vi "Gyro_State_Art.vi"(0 "reset integrator":bool, 1 "[ESC]":bool) -> (6 "Linear Acceleration [LSB/sec^2]":cluster{i16, i16, i16}(graph), 7 "Z displacement":dbl format="%#_5g", 8 "X acc":i16, 9 "Y displacement":dbl format="%#_5g", 10 "Y acc":i16, 11 "X displacement":dbl format="%#_5g", 12 "Angular rate [LSB/sec]":cluster{dbl, dbl, dbl}(graph), 13 "Y rot rate":i16, 14 "Z acc":i16, 15 "Z rot rate":i16, 16 "Temp":i16, 17 "Angular displacement [LSB]":T1(graph), 18 "X rot rate":i16)   [LabVIEW 2017]
uses:
  <vilib>/myRIO/Instrument Drivers/Onboard IO/I2C/typedefs/I2C User Configuration.ctl
  <vilib>/myRIO/Instrument Drivers/Onboard IO/I2C/typedefs/I2C Transfer Rate.ctl
  <vilib>/Platform/TimedLoop/XDataNode/timing_clust.ctl
  <vilib>/Platform/TimedLoop/XDataNode/nitl_modes.ctl
  <vilib>/Platform/TimedLoop/XDataNode/wakeup.ctl
  <vilib>/myRIO/Instrument Drivers/Onboard IO/PWM/typedefs/PWM Reference.ctl
  <vilib>/myRIO/Common/Instrument Driver Framework/Utilities/typedefs/myRIO Generic Hardware Reference.ctl
  <vilib>/myRIO/Common/Instrument Driver Framework/Utilities/typedefs/Hardware Version Enum.ctl
  <vilib>/myRIO/Common/Instrument Driver Framework/Utilities/typedefs/myRIO v1.0 Reference.ctl
  <vilib>/myRIO/Common/Instrument Driver Framework/Utilities/typedefs/Generic FPGA Reference.ctl
  <vilib>/myRIO/Common/Instrument Driver Framework/myRIO v1.0/PWM/typedefs/PWM Channels Enum.ctl
  <vilib>/myRIO/Instrument Drivers/Onboard IO/PWM/typedefs/PWM Configuration.ctl
  <vilib>/userdefined/High Color/nirio_resource_hc.ctl
  <vilib>/myRIO/Common/Instrument Driver Framework/Utilities/vis/Is FPGA Ref Available.vi
  <vilib>/myRIO/Common/Instrument Driver Framework/myRIO v1.0/PWM/vis/myRIO v1.1 Open PWM.vi
  <vilib>/myRIO/Instrument Drivers/Onboard IO/PWM/vis/Set Duty Cycle and Frequency.vi
  <vilib>/myRIO/Common/Instrument Driver Framework/myRIO v1.0/DIO/vis/myRIO v1.1 Open DIO.vi
  <vilib>/myRIO/Common/Instrument Driver Framework/myRIO v1.0/I2C/vis/myRIO v1.1 Open I2C.vi
  <vilib>/myRIO/Common/Instrument Driver Framework/Utilities/vis/Validate Channels.vi
  <vilib>/myRIO/Common/Instrument Driver Framework/myRIO v1.0/PWM/vis/myRIO v1.0 Reserve PWM.vi
  <vilib>/myRIO/Common/Instrument Driver Framework/myRIO v1.0/UART/vis/myRIO v1.0 Close UART.vi
  <vilib>/myRIO/Common/Instrument Driver Framework/myRIO v1.0/DIO/vis/myRIO v1.0 Reserve DIO.vi
  <vilib>/myRIO/Common/Instrument Driver Framework/myRIO v1.0/I2C/vis/myRIO v1.0 Reserve I2C.vi
  <vilib>/myRIO/Common/Instrument Driver Framework/myRIO v1.0/PWM/vis/myRIO v1.0 Build MUX Configuration PWM.vi
  <vilib>/myRIO/Common/Instrument Driver Framework/myRIO v1.0/Resource Manager/vis/myRIO v1.0 Reserve Channel List.vi
  <vilib>/myRIO/Common/Instrument Driver Framework/myRIO v1.0/DIO/vis/myRIO v1.0 Build MUX Configuration DIO.vi
  <vilib>/myRIO/Common/Instrument Driver Framework/myRIO v1.0/I2C/vis/myRIO v1.0 Build MUX Configuration I2C.vi
  <vilib>/myRIO/Common/Instrument Driver Framework/myRIO v1.0/Resource Manager/vis/myRIO v1.0 Create Configuration List.vi
  <vilib>/myRIO/Common/Instrument Driver Framework/myRIO v1.0/Resource Manager/vis/myRIO v1.0 Reserve Channel.vi
  <vilib>/myRIO/Common/Instrument Driver Framework/myRIO v1.0/Resource Manager/vis/myRIO v1.0 Unreserve Channel.vi
  <vilib>/myRIO/Common/Instrument Driver Framework/myRIO v1.0/Resource Manager/vis/myRIO v1.0 Build Mutex Name.vi
  <vilib>/Utility/VariantDataType/GetNumericInfo.vi
  <vilib>/Utility/error.llb/Error Cluster From Error Code.vi
  <vilib>/myRIO/Common/Instrument Driver Framework/myRIO v1.0/myRIO v1.1 Open.vi
  <vilib>/myRIO/Common/Instrument Driver Framework/Utilities/vis/IO Manager.vi
  <vilib>/myRIO/Common/Instrument Driver Framework/Utilities/vis/Configuration Manager.vi
  <vilib>/myRIO/Common/Instrument Driver Framework/myRIO v1.0/Resource Manager/vis/myRIO v1.0 Configure IO.vi
  <vilib>/myRIO/Common/Instrument Driver Framework/myRIO v1.0/myRIO v1.0 Close.vi
  <vilib>/myRIO/Common/Instrument Driver Framework/myRIO v1.0/I2C/vis/myRIO v1.0 Configure I2C.vi
  <vilib>/myRIO/Common/Instrument Driver Framework/myRIO v1.0/I2C/vis/myRIO v1.0 Write I2C.vi
  <vilib>/myRIO/Common/Instrument Driver Framework/myRIO v1.0/PWM/vis/myRIO v1.0 Write PWM.vi
  <vilib>/myRIO/Common/Instrument Driver Framework/myRIO v1.0/DIO/vis/myRIO v1.0 Read DIO.vi
  <vilib>/myRIO/Common/Instrument Driver Framework/myRIO v1.0/I2C/vis/myRIO v1.0 Read I2C.vi
  <vilib>/myRIO/Common/Instrument Driver Framework/Utilities/vis/FPGA Ref Manager.vi
  <vilib>/myRIO/Common/Instrument Driver Framework/myRIO v1.0/myRIO v1.0 Reset FPGA.vi
  <vilib>/myRIO/Common/Instrument Driver Framework/myRIO v1.0/IRQ/vis/myRIO v1.0 IRQ Info FGV.vi
  <vilib>/myRIO/Common/Instrument Driver Framework/myRIO v1.0/IRQ/vis/myRIO v1.0 Timer IRQ Info FGV.vi
  <vilib>/myRIO/Common/Instrument Driver Framework/myRIO v1.0/IRQ/vis/myRIO v1.0 ISR Agent.vi
  <vilib>/Platform/TimedLoop/XDataNode/XDataNode.xnode
  <vilib>/myRIO/Express VI/Onboard IO/PWM/PWM Express VI.xnode
  <vilib>/myRIO/Instrument Drivers/Onboard IO/PWM/vis/myRIO PWM Open.xnode
  <vilib>/myRIO/Instrument Drivers/Utilities/Utilities.lvlib
  <vilib>/myRIO/Instrument Drivers/Onboard IO/I2C/I2C.lvlib
  <vilib>/myRIO/Instrument Drivers/Onboard IO/DIO/DIO.lvlib
  <vilib>/Platform/TimedLoop/XDataNode/XDNodeRunTimeDep.lvlib
  <vilib>/ptbypt/NI_PtbyPt.lvlib
  <vilib>/myRIO/Instrument Drivers/Onboard IO/PWM/PWM.lvlib
panel:
  in  "Brushless controller Duty Cycle":dbl(slide)=0.05 scale=0.05..0.1 scale format="%#_6f"
  in  "Duty Cycle MCC2 : Faixa de operação":dbl(slide) scale=0.0..1.0
  in  "Controle sentido M2":bool
  in  "Duty Cycle MCC1 : Faixa de operação":dbl(slide) scale=0.0..1.0
  in  "Ligar (StandBy)":bool
  in  "Controle sentido M1":bool
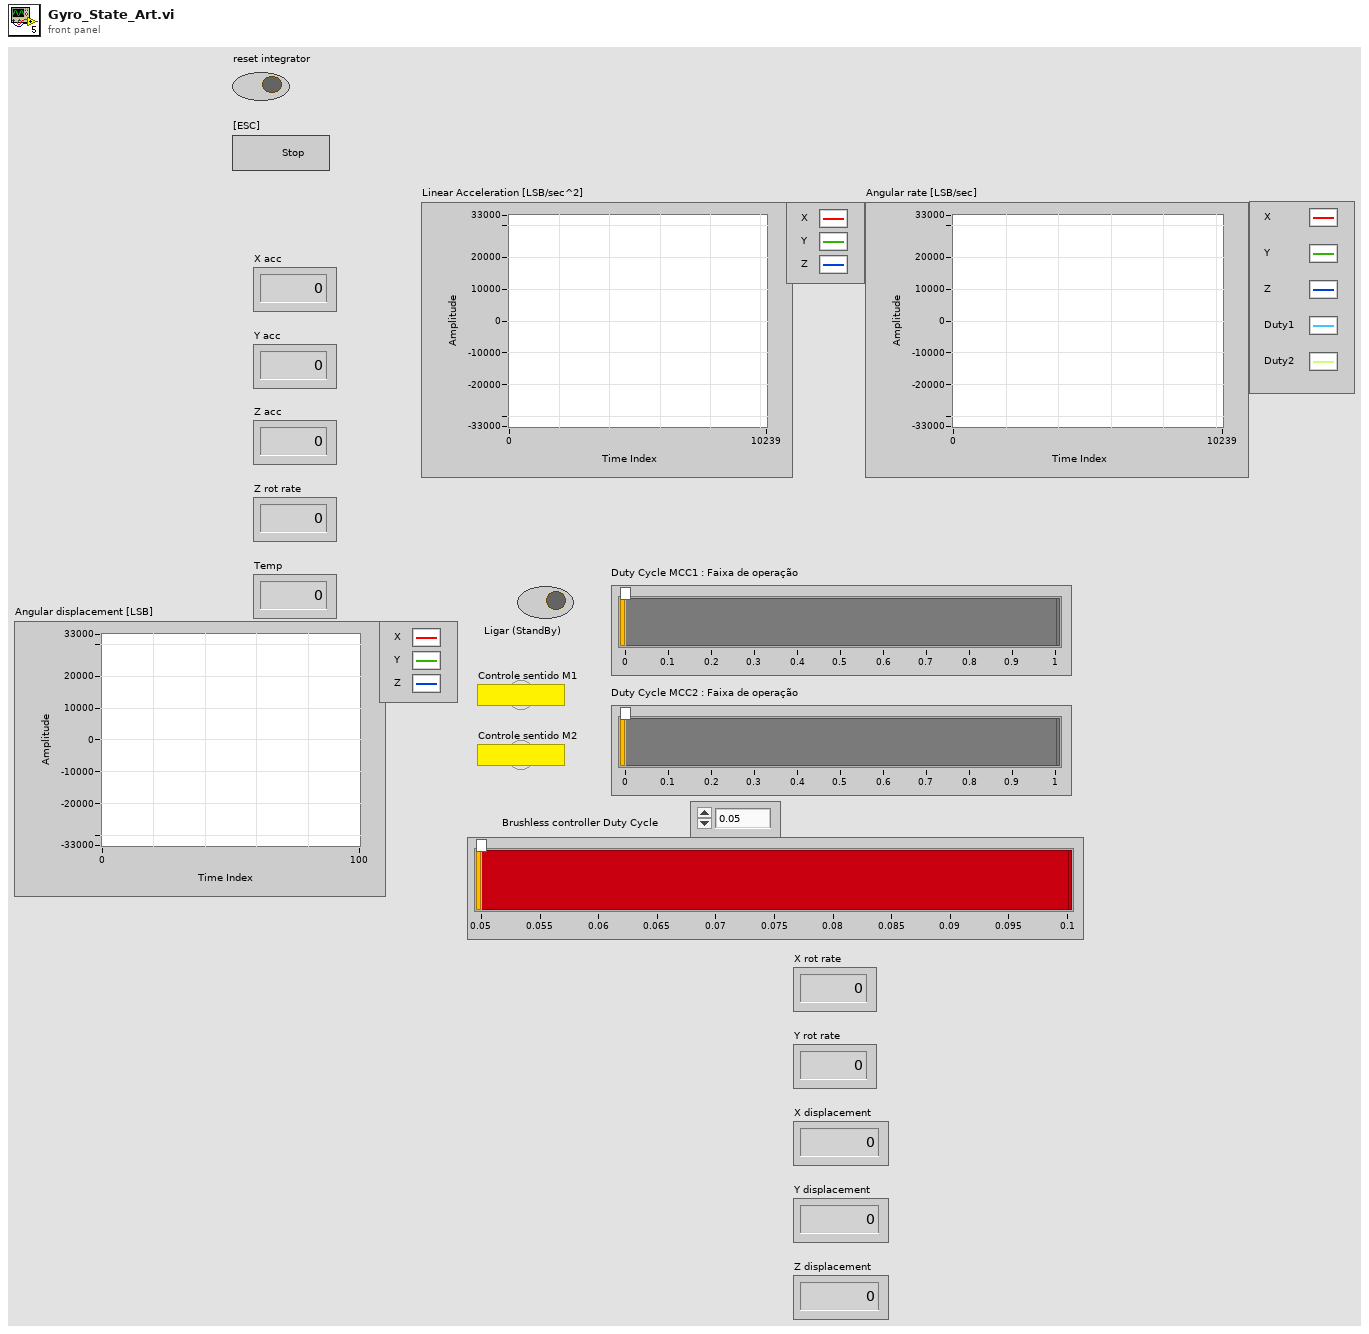
[diagram p1: front panel]
types:
  T1 = cluster{"integral x(t)":dbl, "integral x(t)":dbl, "integral x(t)":dbl}
  T2 = typedef "I2C.lvlib/I2C User Configuration.ctl" = cluster{"I2C Transfer Rate":T3}
  T3 = typedef "I2C.lvlib/I2C Transfer Rate.ctl" = enum16{"Standard mode (100 kbps)", "Fast mode (400 kbps)"}
  T4 = typedef "I2C.lvlib/I2C Reference.ctl" = cluster{"myRIO Reference":T5, "I2C Channels Enum":T9, "I2C Configuration":T10}
  T5 = typedef "myRIO Generic Hardware Reference.ctl" = cluster{"myRIO Model":T6, "myRIO Hardware Reference":T7}
  T6 = typedef "Hardware Version Enum.ctl" = enum16{"Unknown", "myRIO-1900", "myRIO-1950", "roboRIO", "NI ELVIS RIO CM"}
  T7 = typedef "myRIO v1.0 Reference.ctl" = cluster{"Generic FPGA Reference":T8, "Allow multiple opens":bool}
  T8 = typedef "Generic FPGA Reference.ctl" = refnum<k20>
  T9 = typedef "I2C Channels Enum.ctl" = enum16{"Not Connected", "A/I2C", "B/I2C", "I2C/I2C"}
  T10 = typedef "I2C.lvlib/I2C Configuration.ctl" = cluster{"I2C Transfer Rate":T3}
  T11 = typedef "DIO.lvlib/DIO Reference.ctl" = cluster{"myRIO Reference":T5, "DIO Channels List":T12}
  T12 = typedef "DIO Channels List.ctl" = T13[]
  T13 = typedef "DIO Channels Enum.ctl" = enum16{"Not Connected", "C/DIO0", "C/DIO1", "C/DIO2", "C/DIO3", "C/DIO4", "C/DIO5", "C/DIO6", "C/DIO7", "A/DIO0", "A/DIO1", "A/DIO2", "A/DIO3", "A/DIO4", "A/DIO5", "A/DIO6", "A/DIO7", "A/DIO8", "A/DIO9", "A/DIO10", "A/DIO11", "A/DIO12", "A/DIO13", "A/DIO14", "A/DIO15", "B/DIO0", "B/DIO1", "B/DIO2", "B/DIO3", "B/DIO4", "B/DIO5", "B/DIO6", "B/DIO7", "B/DIO8", "B/DIO9", "B/DIO10", "B/DIO11", "B/DIO12", "B/DIO13", "B/DIO14", "B/DIO15", "LED0", "LED1", "LED2", "LED3", "Button0", "DIO/DIO0", "DIO/DIO1", "DIO/DIO2", "DIO/DIO3", "DIO/DIO4", "DIO/DIO5", "DIO/DIO6", "DIO/DIO7", "DIO/DIO8", "DIO/DIO9", "SPI/CS0", "SPI/CS1", "SPI/CS2", "SPI/CS3", "LED RADIO (Green)", "LED RADIO (Red)", "LED COMM (Green)", "LED COMM (Red)", "LED MODE (Green)", "LED MODE (Red)"}
  T14 = typedef "XDNodeRunTimeDep.lvlib/timing_clust.ctl" = cluster{"Expected End [f-1]":u64, "Actual End [f-1]":u64, "Finished Late? [f-1]":bool, "Expected End [i-1]":u64, "Actual End [i-1]":u64, "Finished Late? [i-1]":bool, "Expected Start [i]":u64, "Actual Start [i]":u64, "Expected Start [f]":u64, "Actual Start [f]":u64, "Source Name":string, "Structure Name":string, "Period":i64, "Deadline":i64, "Offset":i64, "Start":i64, "Priority":i32, "Timeout":i32, "Mode":T15, "Wakeup Reason":T16, "Error":errorcluster, "Source Type":string, "Secondary Source Type":string, "Global End Time":u64, "Global Start Time":u64, "Frame Duration":u64, "Iteration Duration":u64, "Assigned CPU":i32, "I/O Scan Engine Mode":u32}
  T15 = typedef "XDNodeRunTimeDep.lvlib/nitl_modes.ctl" = enum32{"No Change", "Process missed periods, maintain original phase", "Discard missed periods, maintain original phase", "Process missed periods, ignore original phase", "Discard missed periods, ignore original phase"}
  T16 = typedef "XDNodeRunTimeDep.lvlib/wakeup.ctl" = enum32{"Normal", "Aborted", "Asynchronous wakeup", "Timing source error", "Timed loop error", "Timeout"}
  T17 = typedef "PWM.lvlib/PWM Reference.ctl" = cluster{"myRIO Reference":T5, "PWM Channels Enum":T18, "PWM Configuration":T19}
  T18 = typedef "PWM Channels Enum.ctl" = enum16{"Not Connected", "C/PWM0", "C/PWM1", "A/PWM0", "A/PWM1", "A/PWM2", "B/PWM0", "B/PWM1", "B/PWM2", "PWM/PWM0", "PWM/PWM1", "PWM/PWM2", "PWM/PWM3", "PWM/PWM4", "PWM/PWM5", "PWM/PWM6", "PWM/PWM7", "PWM/PWM8", "PWM/PWM9"}
  T19 = typedef "PWM.lvlib/PWM Configuration.ctl" = cluster{"Frequency":dbl, "Duty Cycle":dbl}
  T20 = typedef "nirio_resource_hc.ctl" = tag
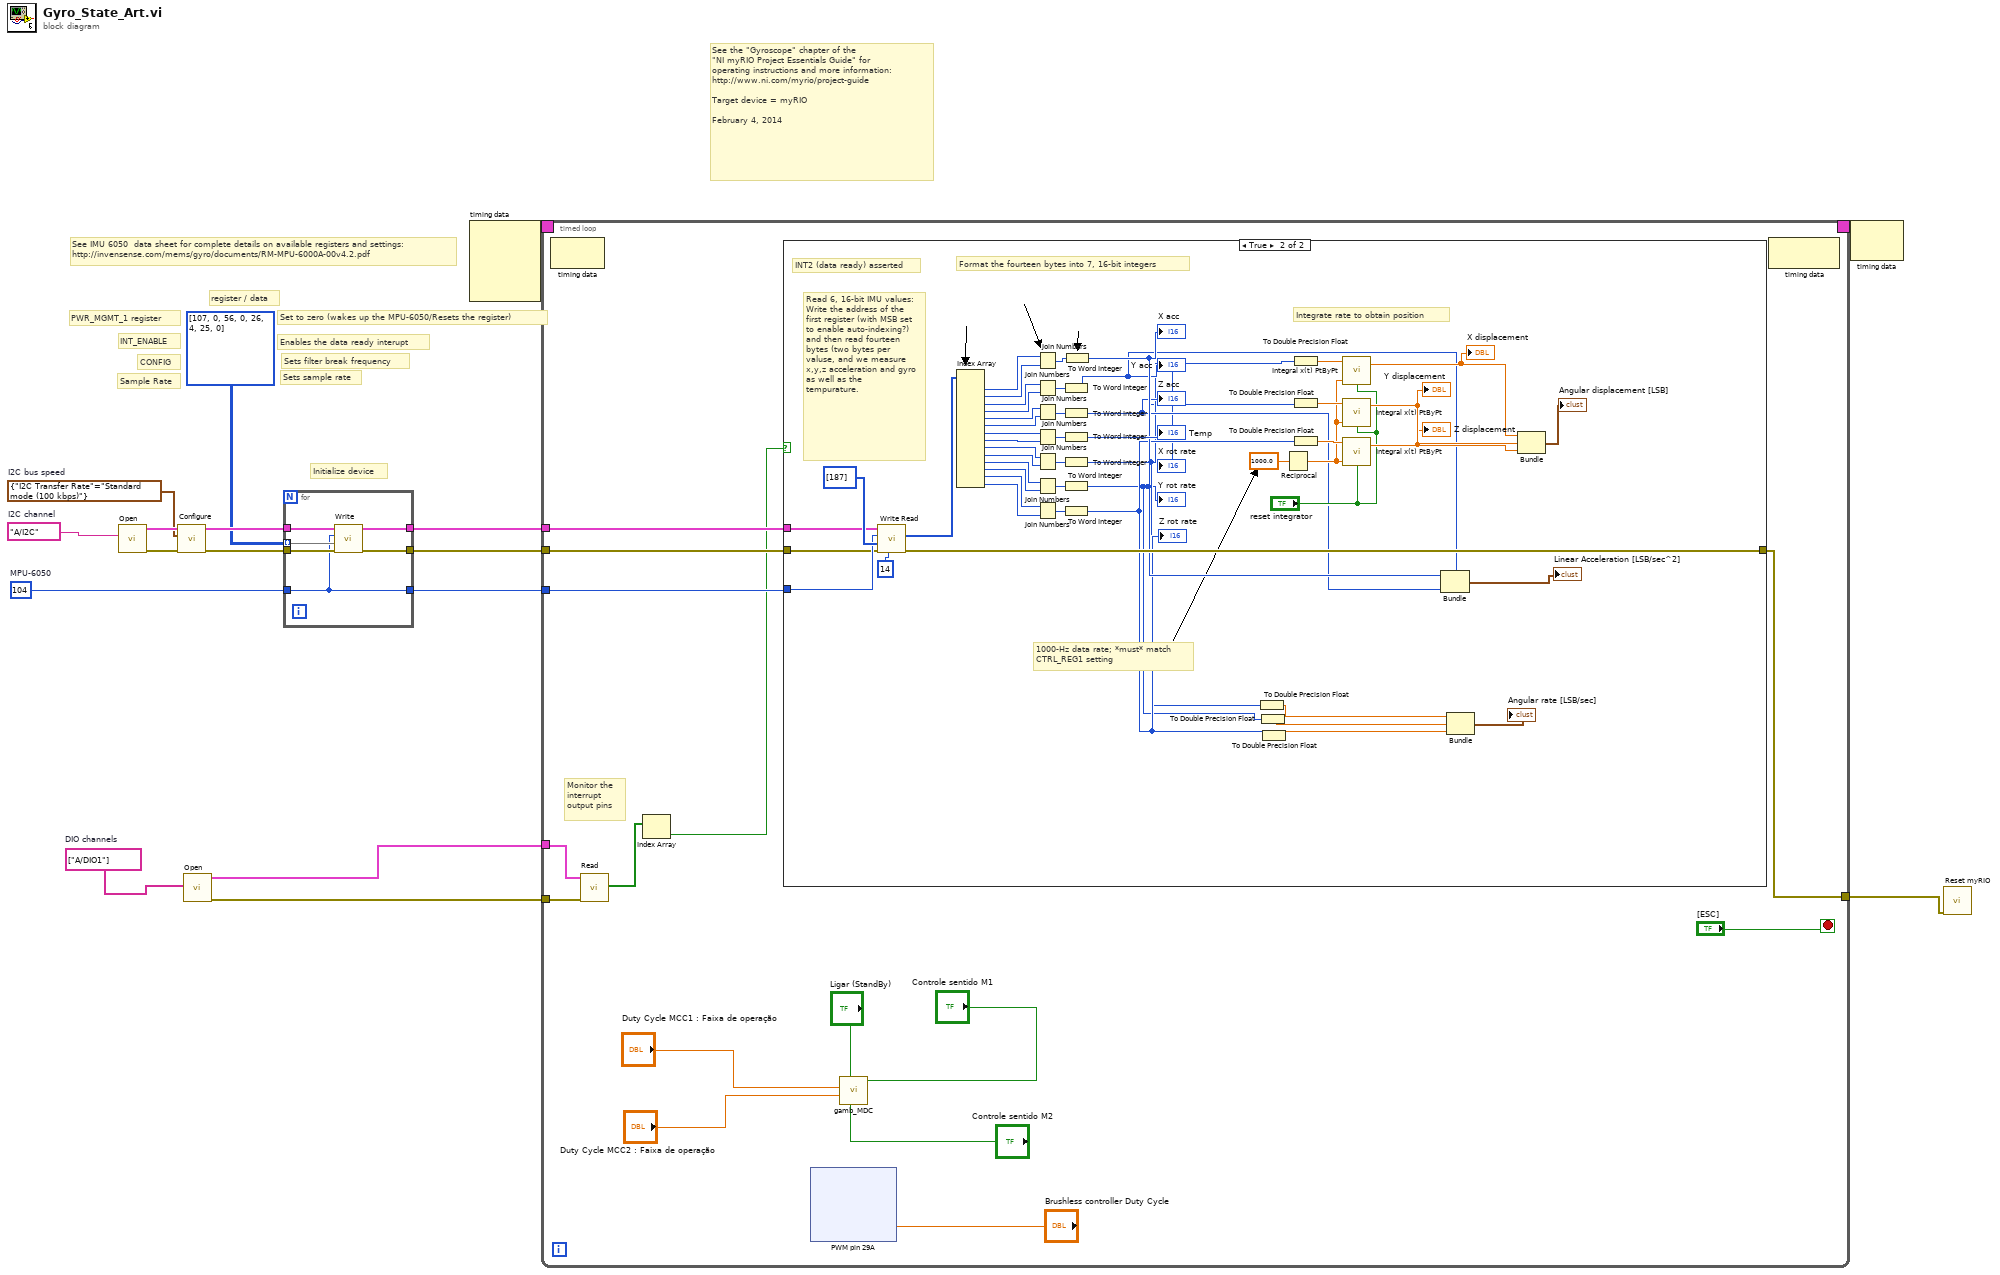
[diagram p0: block diagram]
diagram:
  w13 = tag[] ["A/DIO1"]  # DIO channels
  w2 = T2 {"I2C Transfer Rate"=enum."Standard mode (100 kbps)"}  # I2C bus speed
  w15 = tag "A/I2C"  # I2C channel
  w11 = u8 104  # MPU-6050
  # "Sets sample rate"
  # "Sample Rate"
  # "Sets filter break frequency"
  # "CONFIG"
  # "INT_ENABLE"
  # "Enables the data ready interupt"
  # "See the \"Gyroscope\" chapter of the\n\"NI myRIO Project Essentials Guide\" for\noperating instructions and more information: \nhttp://www.ni.com/myrio/project-guide\n\nTarget device = myRIO\n\nFebruary 4, 2014"
  # "Set to zero (wakes up the MPU-6050/Resets the register)"
  # "PWR_MGMT_1 register"
  # "Initialize device"
  # "See IMU 6050  data sheet for complete details on available registers and settings:\nhttp://invensense.com/mems/gyro/documents/RM-MPU-6000A-00v4.2.pdf"
  # "register / data"
  n1 = call <vilib>:"Open.vi"("Channel Name"=w15) -> ("error out"=w4:errorcluster, "I2C Ref Out"=w3:T4)  [unwired: 9 in]
  n2 = call <vilib>:"Configure.vi"("error in (no error)"=w4, "I2C User Configuration"=w2, "I2C Ref In"=w3) -> ("error out"=w10:errorcluster, "I2C Ref Out"=w9:T4)  [unwired: 7 in]
  n3 = call <vilib>:"Open.vi"("Channel Names"=w13) -> ("error out"=w12:errorcluster, "DIO Ref Out"=w14:T11)  [unwired: 9 in]
  n4 = for {
    tunnel: [w23] -> w5
    tunnel: [w22] -> w6
    tunnel: [w18] -> w7
    tunnel: u8[][] [[107, 0], [56, 0], [26, 4], [25, 0]] ("Bytes to Write") -> [w21] mode=indexing
    tunnel: w9 -> [w20]
    tunnel: w10 -> [w19]
    tunnel: w11 -> [w18]
    n5 = call <vilib>:"Write.vi"("error in (no error)"=w19, "Bytes to Write"=w21, "Slave Address (7-bit)"=w18, "I2C Ref In"=w20) -> ("error out"=w23:errorcluster, "I2C Ref Out"=w22:T4)  [unwired: 6 in]
  }
  n6 = node-c288() -> (w17:T14)  [unwired: 4 in]
  n7 = timed-loop {
    tunnel: [w25] -> w1
    tunnel: w7 -> [w36]
    tunnel: w5 -> [w38]
    tunnel: w6 -> [w37]
    tunnel: w12 -> [w35]
    timing: w17 -> [_]
    timing-out: [_] -> w16
    tunnel: w14 -> [w32]
    stop <- "[ESC]" stop-if-true
    # "Monitor the\ninterrupt\noutput pins"
    n8 = node-c288() -> ()  [unwired: 1 in, 1 out]
    n9 = call <vilib>:"Read.vi"("error in (no error)"=w35, "DIO Ref In"=w32) -> ("Values"=w33:bool[])  [unwired: 7 in, 2 out]
    n10 = Index Array "Index Array"(array=w33) -> (element=w34:bool)  [unwired: 1 in]
    n11 = case shown="True" w34 {
      tunnel: w38 -> [w76 w114]
      tunnel: w37 -> [_ w115]
      tunnel: w36 -> [_ w121]
      tunnel: [w76 w120] -> w25
      frame False {
        # "INT2 (data ready) deasserted"
      }
      frame True {
        # "1000-Hz data rate; *must* match\nCTRL_REG1 setting"
        # "Integrate rate to obtain position"
        # "INT2 (data ready) asserted"
        # "Read 6, 16-bit IMU values:\nWrite the address of the first register (with MSB set to enable auto-indexing?) and then read fourteen bytes (two bytes per valuse, and we measure x,y,z acceleration and gyro as well as the tempurature."
        # "Format the fourteen bytes into 7, 16-bit integers"
        n12 = call <vilib>:"Write Read.vi"("Byte Count"=u32 14, "error in (no error)"=w114, "Bytes to Write"=u8[] [187], "Slave Address (7-bit)"=w121, "I2C Ref In"=w115) -> ("error out"=w120:errorcluster, "Bytes Read"=w119:u8[])  [unwired: 3 in, 1 out]
        n13 = Index Array "Index Array"(array=w119) -> (element #1=w106:u8, element #2=w105:u8, element #3=w104:u8, element #4=w103:u8, element #5=w102:u8, element #6=w101:u8, element #7=w100:u8, element #8=w99:u8, element #9=w98:u8, element #10=w97:u8, element #11=w96:u8, element #12=w95:u8, element #13=w94:u8, element #14=w93:u8)  [unwired: 14 in]
        n14 = Join Numbers(hi=w106, lo=w105) -> ((hi.lo)=w126:u16)
        n15 = Join Numbers(hi=w104, lo=w103) -> ((hi.lo)=w125:u16)
        n16 = Join Numbers(hi=w102, lo=w101) -> ((hi.lo)=w124:u16)
        n17 = Join Numbers(hi=w100, lo=w99) -> ((hi.lo)=w92:u16)
        n18 = Join Numbers(hi=w98, lo=w97) -> ((hi.lo)=w91:u16)
        n19 = Join Numbers(hi=w96, lo=w95) -> ((hi.lo)=w90:u16)
        n20 = Join Numbers(hi=w94, lo=w93) -> ((hi.lo)=w89:u16)
        n21 = To Word Integer(number=w125) -> (16bit integer=w85:i16)
        "Y acc" <- w85
        n22 = To Word Integer(number=w124) -> (16bit integer=w84:i16)
        "Z acc" <- w84
        n23 = To Word Integer(number=w92) -> (16bit integer=→"Temp":i16)
        n24 = To Word Integer(number=w91) -> (16bit integer=w81:i16)
        "X rot rate" <- w81
        n25 = To Word Integer(number=w90) -> (16bit integer=w79:i16)
        "Y rot rate" <- w79
        n26 = To Word Integer(number=w89) -> (16bit integer=w83:i16)
        "Z rot rate" <- w83
        n27 = To Word Integer(number=w126) -> (16bit integer=w86:i16)
        "X acc" <- w86
        n28 = To Double Precision Float(number=w81) -> (double precision float=w80:dbl)
        n29 = To Double Precision Float(number=w79) -> (double precision float=w78:dbl)
        n30 = To Double Precision Float(number=w83) -> (double precision float=w82:dbl)
        n31 = Reciprocal(x=1000.0 ("dt")) -> (1/x=w112:dbl)
        n32 = To Double Precision Float(number=w81) -> (double precision float=w107:dbl)
        n33 = To Double Precision Float(number=w79) -> (double precision float=w118:dbl)
        n34 = To Double Precision Float(number=w83) -> (double precision float=w117:dbl)
        n35 = call <vilib>:"Integral x(t) PtByPt.vi"("initialize"="reset integrator", "dt"=w112, "x"=w107) -> ("integral x(t)"=w108:dbl)  [unwired: 1 in, 1 out]
        "X displacement" <- w108
        n36 = call <vilib>:"Integral x(t) PtByPt.vi"("initialize"="reset integrator", "dt"=w112, "x"=w118) -> ("integral x(t)"=w111:dbl)  [unwired: 1 in, 1 out]
        "Y displacement" <- w111
        n37 = call <vilib>:"Integral x(t) PtByPt.vi"("initialize"="reset integrator", "dt"=w112, "x"=w117) -> ("integral x(t)"=w110:dbl)  [unwired: 1 in, 1 out]
        "Z displacement" <- w110
        n38 = Bundle "Bundle"(w86, w85, w84) -> (→"Linear Acceleration [LSB/sec^2]":cluster{i16, i16, i16})  [unwired: 1 in]
        n39 = Bundle "Bundle"(w80, w78, w82) -> (→"Angular rate [LSB/sec]":cluster{dbl, dbl, dbl})  [unwired: 1 in]
        n40 = Bundle "Bundle"("integral x(t)"=w108, "integral x(t)"=w111, "integral x(t)"=w110) -> (→"Angular displacement [LSB]":T1)  [unwired: 1 in]
      }
    }
    n41 = xnode "PWM pin 29A"("Duty Cycle"="Brushless controller Duty Cycle") -> ()  [unwired: 1 in, 1 out]
    n42 = call "gamb_MDC.vi"("Controle sentido M2"="Controle sentido M2", "Ligar (StandBy)"="Ligar (StandBy)", "Duty Cycle MCC2 : Faixa de operação  in"="Duty Cycle MCC2 : Faixa de operação", "Duty Cycle MCC1 : Faixa de operação in"="Duty Cycle MCC1 : Faixa de operação", "Controle sentido M1"="Controle sentido M1") -> ()  [unwired: 5 in, 2 out]
    n43 = node-c288() -> ()  [unwired: 1 in, 1 out]
  }
  n44 = node-c288(w16) -> ()  [unwired: 1 out]
  n45 = call <vilib>:"Reset myRIO.vi"("error in (no error)"=w1) -> ()  [unwired: 10 in, 1 out]
